vi "Keithley 27XX Totalizer.vi"() -> ()   [LabVIEW 2020]
doc: "This example VI shows how to use the totalizer feature included on the Model 7706 card.\n\nMake sure the front INPUT switch is pushed in (Rear).\n\n\nUse the following steps to Verify the Model 7706 Totalizer function:\n\n1. Connect the function generator to the Model 7706 Totalizer IN+ and IN- terminals\n2. Make sure to leave gate inputs (G+ and G-) open (gate always).\n3. Set the threshold jumper to the TTL position (J2 closed).\n4. Close and lock the Model 7706 Cover.\nNOTE: Make sure the Model 2700 is OFF before installing the Model 7706\n5. Install the Model 7706 in slot 1 of the Model 2700\n6. Turn on the Model 2700\n7. Set the function generator to:\n - Burst mode\n - Burst cycle count of 50,000\n - Manual trigger source\n - Output: 100kHz\n - 0-5V square wave (50% duty cycle)\n8. Enter 125 for 'Totalizer Channel'\n9. Run the VI\n10. Verify that each time the function generator is triggered to output a burst,\n the Totalizer count increases by 50,000"
uses:
  <instrlib>/Keithley 27XX/Keithley 27XX.lvlib
panel:
  in  "Serial Configuration":T1={"Baud Rate (9600)"=9600, "Flow Control (1: XON/XOFF)"=1, "Termination Char (0:CR)"=0} {"Termination Char (0:CR)" items=["CR", "LF"]; "Flow Control (1: XON/XOFF)" items=["None", "XON/XOFF", "RTS/CTS (2701 Only)", "XON/XOFF & RTS/CTS (2701 Only)"]; "Baud Rate (9600)" items=["300"=300, "600"=600, "1200"=1200, "2400"=2400, "4800"=4800, "9600"=9600, "19.2k"=19200, "38.4k (2701 Only)"=38400, "57.6k (2701 Only)"=57600, "115.2k (2701 Only)"=115200]}
  in  "Reset After Read (False)":bool
  in  "Totalizer Channel (125)":string="125"
  in  "VISA resource name":refnum<visa-resource-name>
  out "Totalizer Count":i32
  # "© 2005 National Instruments Corporation.  ALL RIGHTS RESERVED."
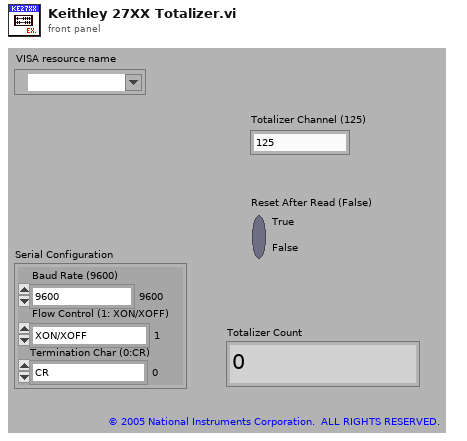
[diagram p1: front panel]
types:
  T1 = cluster{"Baud Rate (9600)":u32, "Flow Control (1: XON/XOFF)":u16, "Termination Char (0:CR)":u16}
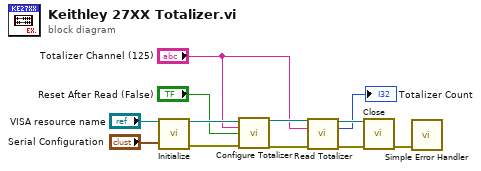
[diagram p0: block diagram]
diagram:
  n1 = call <instrlib>:"Initialize.vi"("VISA resource name"="VISA resource name", "Serial Configuration"="Serial Configuration") -> ("VISA resource name out"=w10:refnum<visa-resource-name>, "error out"=w9:errorcluster)  [unwired: 12 in]
  n2 = call <instrlib>:"Configure Totalizer.vi"("VISA resource name"=w10, "Totalizer Channel (125)"="Totalizer Channel (125)", "Reset After Read (False)"="Reset After Read (False)", "error in (no error)"=w9) -> ("VISA resource name out"=w8:refnum<visa-resource-name>, "error out"=w7:errorcluster)  [unwired: 10 in]
  n3 = call <instrlib>:"Read Totalizer.vi"("VISA resource name"=w8, "Totalizer Channel (125)"="Totalizer Channel (125)", "error in (no error)"=w7) -> ("VISA resource name out"=w5:refnum<visa-resource-name>, "Totalizer Count"=→"Totalizer Count":i32, "error out"=w6:errorcluster)  [unwired: 10 in]
  n4 = call <instrlib>:"Close.vi"("VISA resource name"=w5, "error in (no error)"=w6) -> ("error out"=w11:errorcluster)  [unwired: 13 in]
  n5 = call <vilib>:"Simple Error Handler.vi"("error in (no error)"=w11) -> ()  [unwired: 4 in, 5 out]
